vi "Configure Frequency Sweep.vi"(8 "error in (no error)":errorcluster, 10 "Freq Sweep Setting":T1={"Sweep Spacing (0: Linear)"=0, "Sweep Time (1.00 s)"=1.0, "Stop  Frequency (1000.0 Hz)"=1000.0, "Start Frequency (100.0 Hz)"=100.0, "Enable/Disable Freq Sweep"=FALSE} {"Start Frequency (100.0 Hz)" format="%#.6g"; "Stop  Frequency (1000.0 Hz)" format="%#.6g"; "Sweep Time (1.00 s)" format="%#.6g"; "Sweep Spacing (0: Linear)" items=["Linear", "Logarithmic"]}, 11 "Agilent 33210A in":refnum<class "Agilent 33210A.lvclass">) -> (0 "error out":errorcluster, 3 "Agilent 33210A out":refnum<class "Agilent 33210A.lvclass">)   [LabVIEW 2021, in "Func Generator.lvlib" / "Agilent 33210A.lvclass"]
uses:
  Agilent 33210A.lvclass
  Agilent 33210A.lvclass/Agilent 33210A.ctl
  <instrlib>/Agilent 33XXX Series/Agilent 33XXX Series.lvlib
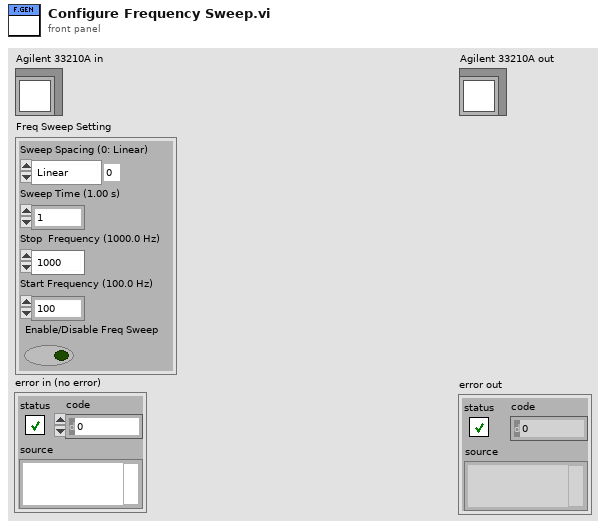
[diagram p1: front panel]
types:
  T1 = cluster{"Sweep Spacing (0: Linear)":u16, "Sweep Time (1.00 s)":dbl, "Stop  Frequency (1000.0 Hz)":dbl, "Start Frequency (100.0 Hz)":dbl, "Enable/Disable Freq Sweep":bool}
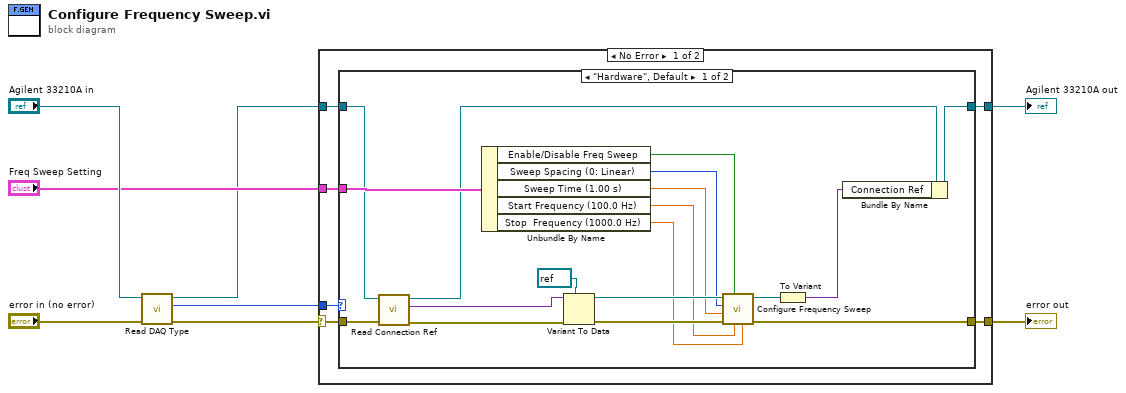
[diagram p0: block diagram]
diagram:
  n1 = call-dynamic "Read DAQ Type.vi"("error in (no error)"="error in (no error)", "Agilent 33210A in"="Agilent 33210A in") -> ("error out"=w7:errorcluster, "DAQ Type"=w6:enum16{"Hardware", "Simulation"}, "Agilent 33210A out"=w1:refnum<class "Agilent 33210A.lvclass">)  [unwired: 7 in]
  n2 = case shown="No Error" w7 {
    selector: w7 -> [w11 w35]
    tunnel: w6 -> [w14 _]
    tunnel: [w13 w36] -> w5
    tunnel: w1 -> [w12 w36]
    tunnel: [w10 w35] -> w3
    tunnel: "Freq Sweep Setting" -> [w9 _]
    frame No Error {
      n3 = case shown="\"Hardware\", Default" w14 {
        tunnel: [w26 w34] -> w13
        tunnel: w12 -> [w16 w34]
        tunnel: w11 -> [w32 w33]
        tunnel: [w24 w33] -> w10
        tunnel: w9 -> [w23 _]
        frame "Hardware", Default {
          n4 = call-dynamic "Read Connection Ref.vi"("error in (no error)"=w32, "Agilent 33210A in"=w16) -> ("error out"=w31:errorcluster, "Connection Ref"=w30:variant, "Agilent 33210A out"=w15:refnum<class "Agilent 33210A.lvclass">)  [unwired: 7 in]
          n5 = Unbundle By Name(w23) -> ("Enable/Disable Freq Sweep"=w22:bool, "Sweep Spacing (0: Linear)"=w21:u16, "Sweep Time (1.00 s)"=w20:dbl, "Start Frequency (100.0 Hz)"=w19:dbl, "Stop  Frequency (1000.0 Hz)"=w18:dbl)
          n6 = Variant To Data(error in=w31, type=refnum<visa-resource-name> refnum ("VISA resource name"), Variant=w30) -> (data=w28:refnum<visa-resource-name>, error out=w27:errorcluster)
          n7 = call <instrlib>:"Configure Frequency Sweep.vi"("Stop  Frequency (1000.0 Hz)"=w18, "Start Frequency (100.0 Hz)"=w19, "Enable Frequency Sweep Mode (T: Enable)"=w22, "error in (no error)"=w27, "Sweep Time (1.00 s)"=w20, "Sweep Spacing (0: Linear)"=w21, "VISA resource name"=w28) -> ("error out"=w24:errorcluster, "VISA resource name out"=w25:refnum<visa-resource-name>)  [unwired: 3 in]
          n8 = To Variant(anything=w25) -> (Variant=w17:variant)
          n9 = Bundle By Name(cluster=w15, "Connection Ref"=w17) -> (w26:refnum<class "Agilent 33210A.lvclass">)
        }
        frame "Simulation" {
        }
      }
    }
    frame Error {
    }
  }
  "error out" <- w3
  "Agilent 33210A out" <- w5
